vi "CheezyAsin.vi"(1 "arg":dbl) -> (0 "asin(arg)":dbl)   [LabVIEW 2015]
uses:
  <userlib>/836-Library/CheezyMath/MathConstantsNames.ctl
panel:
  out "Time to Run":dbl
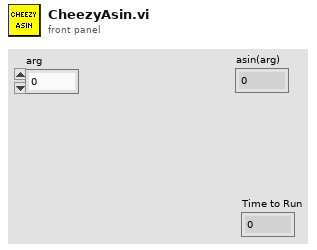
[diagram p1: front panel]
types:
  T1 = typedef "MathConstantsNames.ctl" = enum16{"sq2p1", "sq2m1", "p4", "p3", "p2", "p1", "p0", "q4", "q3", "q2", "q1", "q0", "PIO2"}
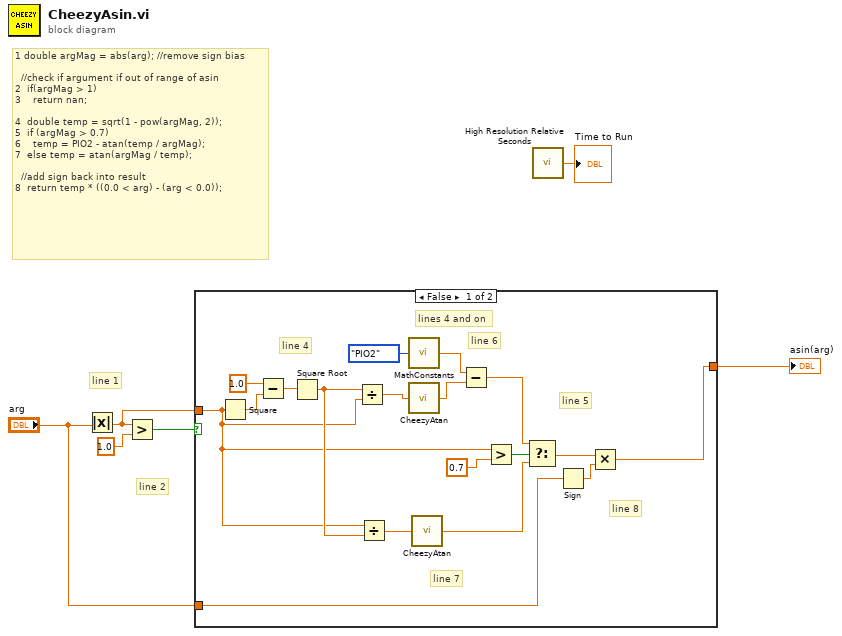
[diagram p0: block diagram]
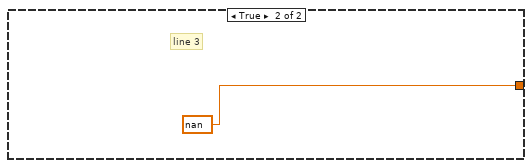
[diagram p2: hidden frame]
diagram:
  # "line 2"
  # "line 1"
  # "1 double argMag = abs(arg); //remove sign bias\n\n  //check if argument if out of range of asin\n2  if(argMag > 1)\n3    return nan;\n\n4  double temp = sqrt(1 - pow(argMag, 2));\n5  if (argMag > 0.7)\n6    temp = PIO2 - atan(temp / argMag);\n7  else temp = atan(argMag / temp);\n  \n  //add sign back into result\n8  return temp * ((0.0 < arg) - (arg < 0.0));"
  n1 = Absolute Value(x="arg") -> (abs(x)=w3:dbl)
  n2 = Greater?(x=w3, y=1.0) -> (0:w6:bool)
  n3 = case shown="False" w6 {
    tunnel: [w7 nan] -> w4
    tunnel: w3 -> [w12 _]
    tunnel: "arg" -> [w8 _]
    frame False {
      # "line 8"
      # "line 6"
      # "line 7"
      # "line 5"
      # "line 4"
      # "lines 4 and on"
      n4 = Square(x=w12) -> (x^2=w22:dbl)
      n5 = Subtract(x=1.0, y=w22) -> (x-y=w24:dbl)
      n6 = Square Root(x=w24) -> (sqrt(x)=w20:dbl)
      n7 = Divide(x=w20, y=w12) -> (x/y=w19:dbl)
      n8 = Divide(x=w12, y=w20) -> (x/y=w18:dbl)
      n9 = call <userlib>:"MathConstants.vi"("Constant Name"=MathConstantsNames."PIO2") -> ("Constant Value"=w17:dbl)
      n10 = call <userlib>:"CheezyAtan.vi"("arg"=w19) -> ("atan(arg)"=w16:dbl)
      n11 = call <userlib>:"CheezyAtan.vi"("arg"=w18) -> ("atan(arg)"=w15:dbl)
      n12 = Subtract(x=w17, y=w16) -> (x-y=w14:dbl)
      n13 = Greater?(x=w12, y=0.7) -> (0:w13:bool)
      n14 = Select(t=w14, s=w13, f=w15) -> (s? t:f=w10:dbl)
      n15 = Sign(1:w8) -> (0:w9:dbl)
      n16 = Multiply(x=w10, y=w9) -> (x*y=w7:dbl)
    }
    frame True {
      # "line 3"
    }
  }
  "asin(arg)" <- w4
  n17 = call <vilib>:"High Resolution Relative Seconds.vi"() -> ("relative seconds"=→"Time to Run":dbl)
